vi "egg_incubator.vi"() -> ()   [LabVIEW 2020]
uses:
  <vilib>/Instr/_visa.llb/VISA Configure Serial Port (Instr).vi
panel:
  in  "?":enum32{"Information ", "Graph   2"}(tab)
  in  "?":bool
  out "?":dbl
  out "?":dbl
  in  "?":refnum<visa-resource-name>
  out "FTR":bool
  out "STR":bool
  out "DR":bool
  out "Temperature Chart":dbl(graph)
  out "Humidity Chart":dbl(graph)
  out "Humidity":dbl(slide) scale=0.0..100.0
  out "Temperature":dbl(slide) scale=0.0..100.0
  # "H"
  # "T"
  # "FTR = Fatal Temperature Range"
  # "DR = Dangerous Range"
  # "STR = Safe Temperature Range"
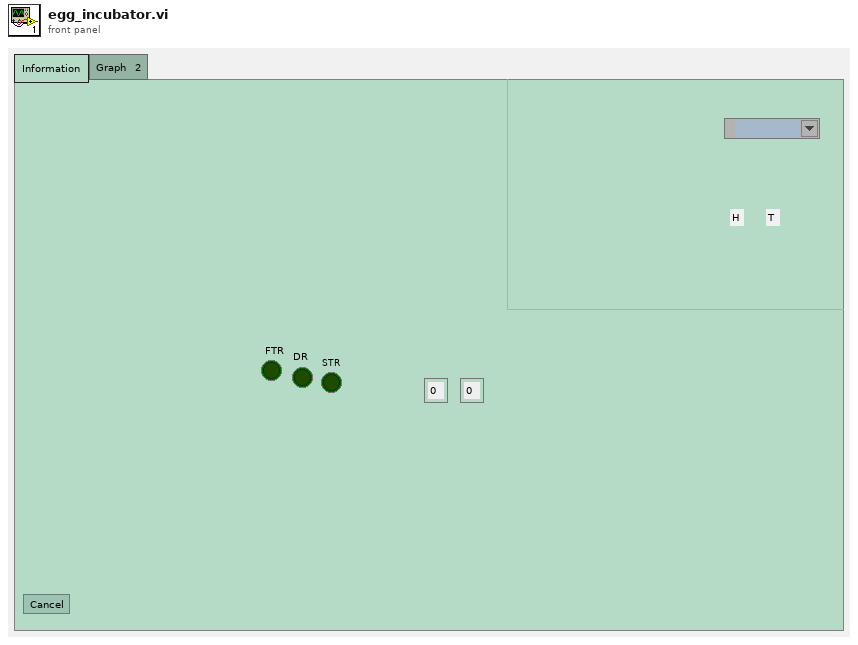
[diagram p1: front panel]
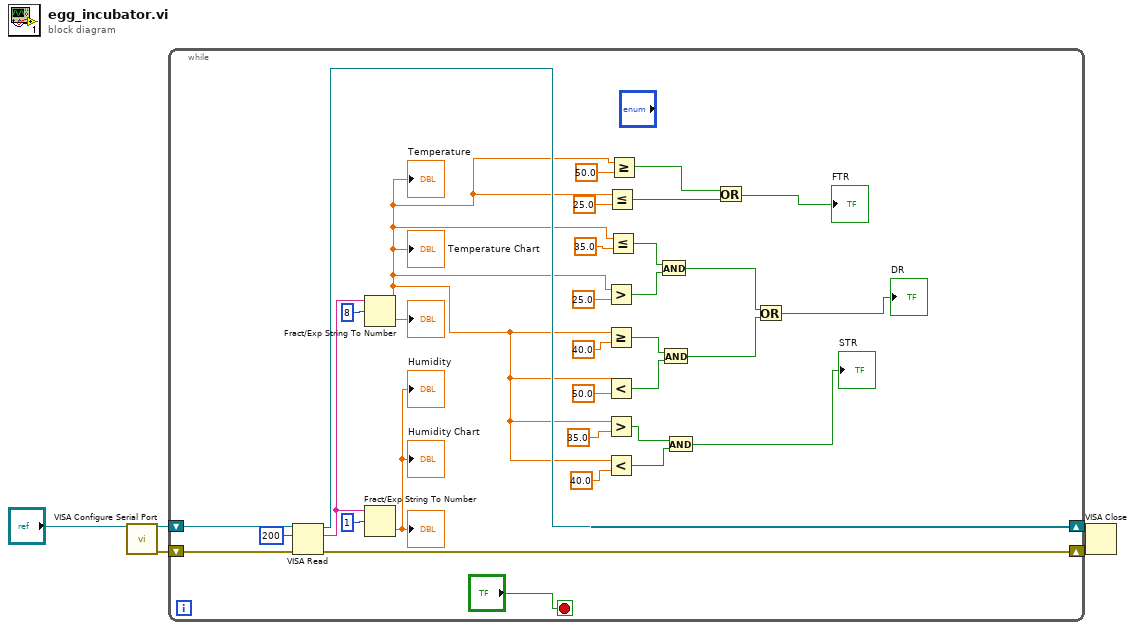
[diagram p0: block diagram]
diagram:
  n1 = call-poly "VISA Configure Serial Port"("VISA resource name"="?") -> ("VISA resource name out"=w4:refnum<visa-resource-name>, "error out"=w3:errorcluster)  [unwired: 13 in]
  n2 = while {
    shift-right: [w37] -> w2
    shift-left: w4 -> [w15]
    shift-right: [w36] -> w1
    shift-left: w3 -> [w14]
    stop <- "?" stop-if-true
    n3 = VISA Read(VISA resource name=w15, byte count=u32 200, error in (no error)=w14) -> (VISA resource name out=w37:refnum<visa-resource-name>, read buffer=w34:string, error out=w36:errorcluster)  [unwired: 1 out]
    n4 = Fract/Exp String To Number(string=w34, offset=8) -> (number=w7:dbl)  [unwired: 2 in, 1 out]
    "?" <- w7
    "Temperature" <- w7
    "Temperature Chart" <- w7
    n5 = Fract/Exp String To Number(string=w34, offset=1) -> (number=→"?" →"Humidity" →"Humidity Chart":dbl)  [unwired: 2 in, 1 out]
    n6 = Greater?(x=w7, y=25.0) -> (0:w23:bool)
    n7 = Greater Or Equal?(x=w7, y=40.0) -> (x >= y?=w21:bool)
    n8 = Less?(x=w7, y=50.0) -> (x < y?=w20:bool)
    n9 = Greater?(x=w7, y=35.0) -> (0:w18:bool)
    n10 = Less?(x=w7, y=40.0) -> (x < y?=w17:bool)
    n11 = Less Or Equal?(x=w7, y=25.0) -> (x <= y?=w11:bool)
    n12 = Less Or Equal?(x=w7, y=35.0) -> (x <= y?=w24:bool)
    n13 = Greater Or Equal?(x=w7, y=50.0) -> (x >= y?=w12:bool)
    n14 = And(x=w24, y=w23) -> (x .and. y?=w22:bool)
    n15 = And(x=w21, y=w20) -> (x .and. y?=w19:bool)
    n16 = And(x=w18, y=w17) -> (x .and. y?=→"STR":bool)
    n17 = Or(x=w12, y=w11) -> (x .or. y?=→"FTR":bool)
    n18 = Or(x=w22, y=w19) -> (x .or. y?=→"DR":bool)
  }
  n19 = VISA Close(VISA resource name=w2, error in (no error)=w1) -> ()  [unwired: 1 out]
